vi "Untitled 4 (SubVI).vi"() -> (1 "New Image 2":T1, 2 "New Image 3":T1, 3 "Refnum out":T1, 4 "New Image":T1)   [LabVIEW 2011, in "MagAnalysis_Online.lvclass"]
uses:
  MagAnalysis_Online.lvclass
  IMAQ Image.ctl
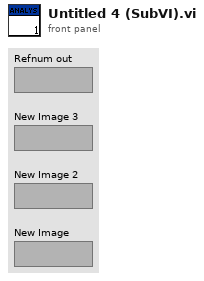
[diagram p1: front panel]
types:
  T1 = typedef "IMAQ Image.ctl" = refnum<image>
  T2 = typedef "Image Type" = u32
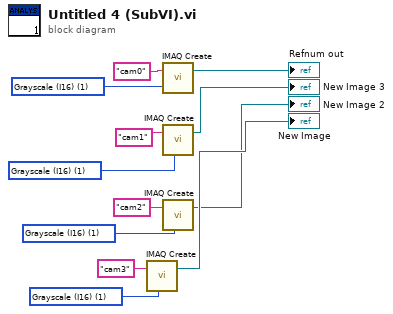
[diagram p0: block diagram]
diagram:
  w10 = T2 1 items=["Grayscale (U8)", "Grayscale (I16)", "Grayscale (SGL)", "Complex (CSG)", "RGB (U32)", "HSL (U32)", "RGB (U64)", "Grayscale (U16)"] ("Image Type")
  w8 = T2 1 items=["Grayscale (U8)", "Grayscale (I16)", "Grayscale (SGL)", "Complex (CSG)", "RGB (U32)", "HSL (U32)", "RGB (U64)", "Grayscale (U16)"] ("Image Type")
  w4 = T2 1 items=["Grayscale (U8)", "Grayscale (I16)", "Grayscale (SGL)", "Complex (CSG)", "RGB (U32)", "HSL (U32)", "RGB (U64)", "Grayscale (U16)"] ("Image Type")
  w2 = T2 1 items=["Grayscale (U8)", "Grayscale (I16)", "Grayscale (SGL)", "Complex (CSG)", "RGB (U32)", "HSL (U32)", "RGB (U64)", "Grayscale (U16)"] ("Image Type")
  n1 = call "IMAQ Create"("Image Name"="cam3", "Image Type"=w10) -> ("New Image"=→"New Image":T1)  [unwired: 3 in, 1 out]
  n2 = call "IMAQ Create"("Image Name"="cam0", "Image Type"=w2) -> ("New Image"=→"Refnum out":T1)  [unwired: 3 in, 1 out]
  n3 = call "IMAQ Create"("Image Name"="cam1", "Image Type"=w4) -> ("New Image"=→"New Image 3":T1)  [unwired: 3 in, 1 out]
  n4 = call "IMAQ Create"("Image Name"="cam2", "Image Type"=w8) -> ("New Image"=→"New Image 2":T1)  [unwired: 3 in, 1 out]
